vi "Execute.vi"(8 "error in (no error)":errorcluster, 9 "Consumer Queues in":T2, 10 "Trig Process Command in":refnum<class "Config and Run TRIG Process.lvclass">, 11 "Trig Process Data in":T1) -> (0 "error out":errorcluster, 1 "Consumer Queues out":T2, 2 "Stop?":bool, 3 "Trig Process Data out":T1)   [LabVIEW 2019, in "Trig Process.lvlib" / "Config and Run TRIG Process.lvclass"]
uses:
  Config and Run TRIG Process.lvclass
  TS Framework/Consumer Queues.ctl
  UI Process/Generic UI Command/Generic UI Process Command.lvclass
  DAC Process/Generic DAC Command/Generic DAC Process Command.lvclass
  Generic Trig Command/Generic Trig Process Command.lvclass
  Trig Process Data.ctl
  Config and Run TRIG Process.lvclass/Config and Run TRIG Process.ctl
  TRIG Next Acq Request/TRIG Next Acq Request.lvclass
  TS Framework/TS Framework.lvlib
  Trig Process.lvlib
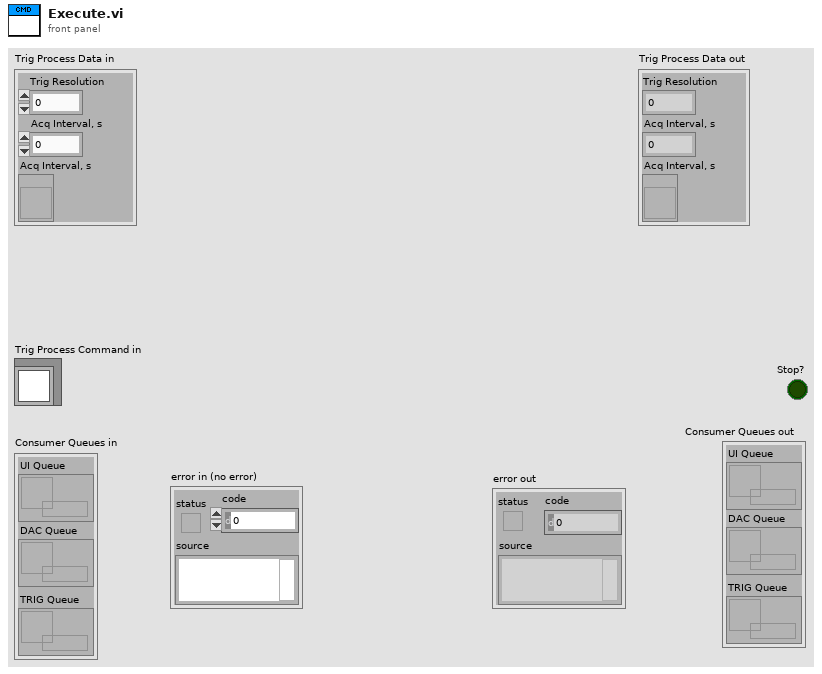
[diagram p1: front panel]
types:
  T1 = typedef "Trig Process.lvlib/Trig Process Data.ctl" = cluster{"Trig Resolution":u32, "Ctrl Interval":dbl, "Acq Interval":refnum<vi>}
  T2 = typedef "TS Framework.lvlib/Consumer Queues.ctl" = cluster{"UI Queue":refnum<queue>, "DAC Queue":refnum<queue>, "TRIG Queue":refnum<queue>}
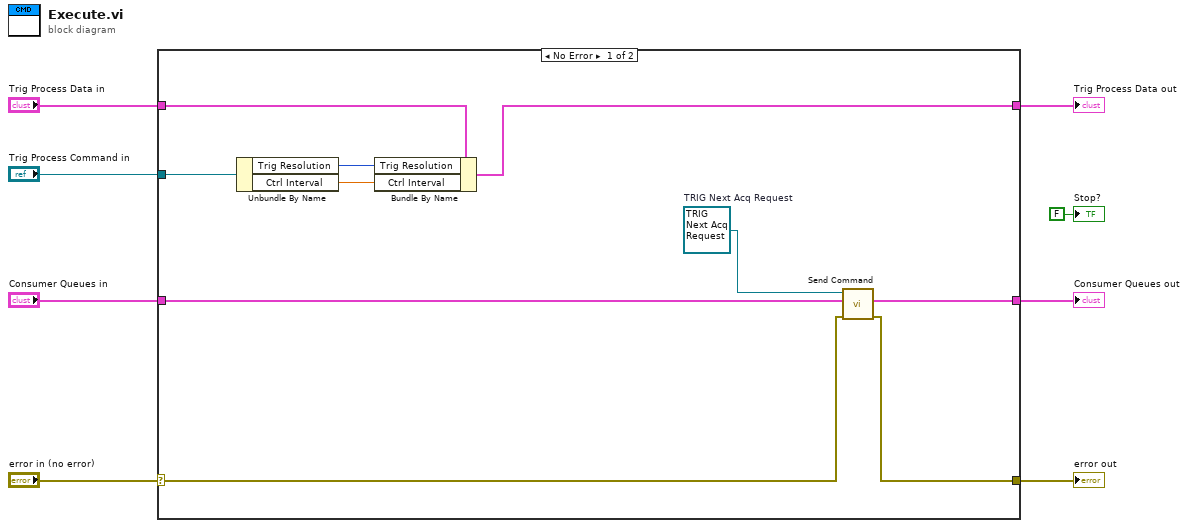
[diagram p0: block diagram]
diagram:
  n1 = case shown="No Error" "error in (no error)" {
    selector: "error in (no error)" -> [w10 w21]
    tunnel: [w9 w21] -> w3
    tunnel: "Consumer Queues in" -> [w13 w20]
    tunnel: [w12 w20] -> w4
    tunnel: "Trig Process Data in" -> [w17 w19]
    tunnel: [w16 w19] -> w5
    tunnel: "Trig Process Command in" -> [w18 _]
    frame No Error {
      w11 = refnum<class "TRIG Next Acq Request.lvclass"> refnum  # TRIG Next Acq Request
      n2 = Unbundle By Name(w18) -> ("Trig Resolution"=w15:u32, "Ctrl Interval"=w14:dbl)
      n3 = Bundle By Name(cluster=w17, "Trig Resolution"=w15, "Ctrl Interval"=w14) -> (w16:T1)
      n4 = call-dynamic "Send Command.vi"("error in (no error)"=w10, "Consumer Queues in"=w13, "Trig Process Command"=w11) -> ("error out"=w9:errorcluster, "Consumer Queues out"=w12:T2)  [unwired: 7 in]
    }
    frame Error {
    }
  }
  "error out" <- w3
  "Consumer Queues out" <- w4
  "Trig Process Data out" <- w5
  "Stop?" <- FALSE ("Stop?")
